vi "Init Action Data.vi"(8 "Motor Labels":string[](array[string]), 9 "Action List":T2(array[cluster])=[{"Action Name"="Enable Motor", "JSON info"=[{"path"="Index", "data type"=enum."INT"}], "String Format"="%(Action Name) %(Index)"}, {"Action Name"="Disable Motor", "JSON info"=[{"path"="Index", "data type"=enum."INT"}], "String Format"="%(Action Name) %(Index)"}, {"Action Name"="Move Motor", "JSON info"=[{"path"="Index", "data type"=enum."INT"}, {"path"="Destination", "data type"=enum."DBL"}], "String Format"="%(Action Name) %(Index) to %(Destination)"}], 10 "Action Data (JSON)":string, 11 "Action Name":string) -> (2 "Data Types":T1(array[cluster]), 3 "Data Names&Defaults":string[][](array[string]))   [LabVIEW 2016, in "Hardware.lvlib" / "Motions.lvlib" / "Motions.lvclass"]
uses:
  <userlib>/Common Components/Hardware/Abstract System/Motions/Motions/Motions.lvclass
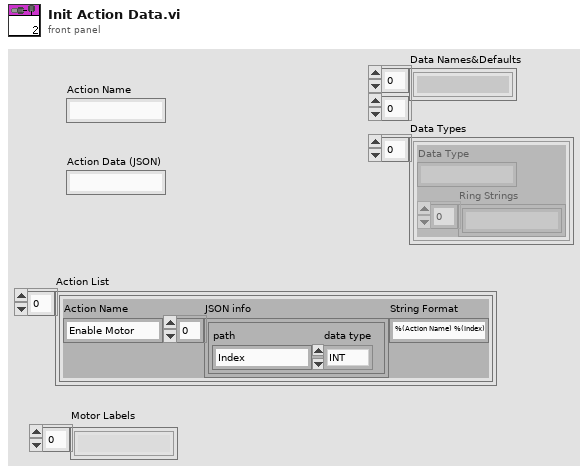
[diagram p1: front panel]
types:
  T1 = cluster{"Data Type":string, "Ring Strings":string[]}[]
  T2 = cluster{"Action Name":string, "JSON info":cluster{"path":string, "data type":enum16{"INT", "DBL", "BOOL", "String"}}[], "String Format":string}[]
  T3 = cluster{"Action Name":string, "JSON info":cluster{"path":string, "data type":enum16{"INT", "DBL", "BOOL", "String"}}[], "String Format":string}
  T4 = cluster{"path":string, "data type":enum16{"INT", "DBL", "BOOL", "String"}}[]
  T5 = cluster{"Data Type":string, "Captioned/Ring Strings":string[]}
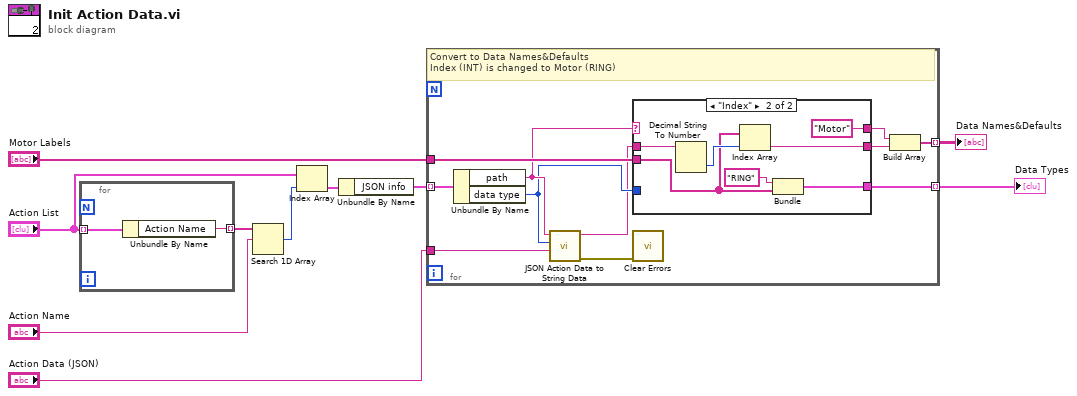
[diagram p0: block diagram]
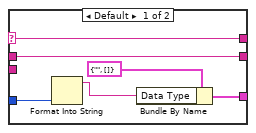
[diagram p2: hidden frame]
diagram:
  n1 = for {
    tunnel: "Action List" -> [w12] mode=indexing
    tunnel: [w11] -> w10 mode=indexing
    n2 = Unbundle By Name(w12) -> ("Action Name"=w11:string)
  }
  n3 = Search 1D Array(1D array=w10, element="Action Name") -> (index of element=w9:i32)  [unwired: 1 in]
  n4 = Index Array(array="Action List", index=w9) -> (element=w7:T3)
  n5 = Unbundle By Name(w7) -> ("JSON info"=w1:T4)
  n6 = for {
    tunnel: w1 -> [w23] mode=indexing
    tunnel: [w19] -> w6 mode=indexing
    tunnel: "Motor Labels" -> [w22]
    tunnel: [w21] -> w5 mode=indexing
    tunnel: "Action Data (JSON)" -> [w16]
    # "Convert to Data Names&Defaults\nIndex (INT) is changed to Motor (RING)"
    n7 = Unbundle By Name(w23) -> ("path"=w18:string, "data type"=w17:enum16{"INT", "DBL", "BOOL", "String"})
    n8 = call <userlib>:"JSON Action Data to String Data.vi"("Action Data (JSON)"=w16, "data type"=w17, "path"=w18) -> ("error out"=w13:errorcluster, "String"=w15:string)  [unwired: 7 in]
    n9 = case shown="\"Index\"" w18 {
      selector: w18 -> [w26 _]
      tunnel: [w26 "Motor" ("element")] -> w20
      tunnel: w22 -> [_ w31]
      tunnel: [w27 w35] -> w21
      tunnel: w17 -> [w25 _]
      tunnel: w15 -> [w24 w33]
      tunnel: [w24 w30] -> w14
      frame Default {
        n10 = Format Into String(w25) -> (resulting string=w28:string)  [unwired: 3 in, 1 out]
        n11 = Bundle By Name(cluster=T5 {"Data Type"="", "Captioned/Ring Strings"=[]}, "Data Type"=w28) -> (w27:T5)
      }
      frame "Index" {
        n12 = Decimal String To Number(string=w33) -> (number=w32:i32)  [unwired: 2 in, 1 out]
        n13 = Index Array(array=w31, index=w32) -> (element=w30:string)
        n14 = Bundle("RING", "Motor Labels"=w31) -> (w35:cluster{string, "Motor Labels":string[]})  [unwired: 1 in]
      }
    }
    n15 = call <vilib>:"Clear Errors.vi"("error in (no error)"=w13) -> ()  [unwired: 5 in, 2 out]
    n16 = Build Array(w20, w14) -> (w19:string[])
  }
  "Data Names&Defaults" <- w6
  "Data Types" <- w5
